vi "Linear Scaling.vi"(1 "Scaling Properties":T1 {"Vmax" min=-10.0 max=10.0 step=1.0; "Vmin" min=-10.0 max=10.0 step=1.0}, 2 "x":dbl) -> (0 "y":dbl)   [LabVIEW 2018]
panel:
  # "y=ax+b"
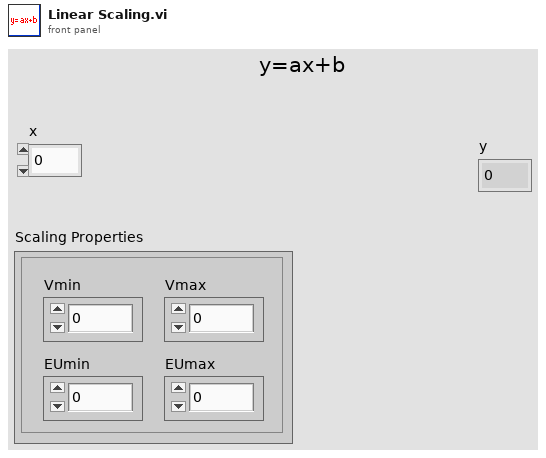
[diagram p1: front panel]
types:
  T1 = cluster{"Vmin":dbl, "Vmax":dbl, "EUmin":dbl, "EUmax":dbl}
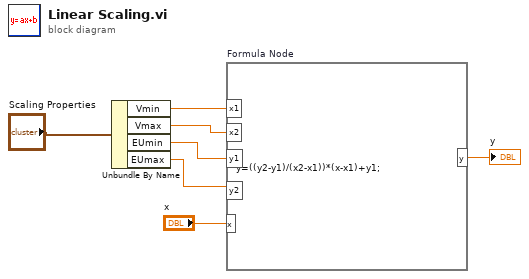
[diagram p0: block diagram]
diagram:
  n1 = Unbundle By Name "Unbundle By Name"("Scaling Properties") -> ("Vmin"=w5:dbl, "Vmax"=w4:dbl, "EUmin"=w3:dbl, "EUmax"=w2:dbl)
  n2 = formula code="y=((y2-y1)/(x2-x1))*(x-x1)+y1;"("x1"=w5, "y1"=w3, "x2"=w4, "y2"=w2, "x"="x") -> ("y"=→"y":dbl)
